vi "SendDrivingCAN.vi"(8 "error in (no error)":errorcluster, 11 "interface object in":refnum<k20>) -> (0 "error out":errorcluster, 3 "interface object out":refnum<k20>)   [LabVIEW 2014]
uses:
  <vilib>/RioEmbeddedCAN/RioEmbeddedCAN.llb/CANFrameControl.ctl
  <vilib>/RioEmbeddedCAN/RioEmbeddedCAN.llb/CANWaitTransmitComplete.vi
  Global Data.vi
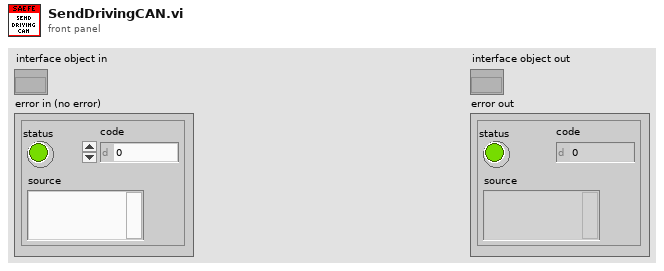
[diagram p1: front panel]
types:
  T1 = typedef "CANFrameControl.ctl" = cluster{"identifier":u32, "extended?":bool, "type":u8, "payload":u8[]}
  T2 = typedef "Lap Statistics.ctl" = cluster{"rBrakeBalLast":dbl}
  T3 = typedef "MC Temp 2.ctl" = cluster{"TMCControlBoard":dbl, "TMCRTD1":dbl, "TMCRTD2":dbl, "TMCRTD3":dbl}
  T4 = typedef "BMS Telemetry.ctl" = cluster{"bBMSIgnition":bool, "bBMSChargerMains":bool, "bBMSFastCharge":bool, "bBMSChargerEnabled":bool, "eBMSCarState":enum16{"Off", "On, Not Charging", "Charging", "Charging Finished", "Charging Error"}, "eBMSChargingState":enum16{"Disconnected", "Pre-charging", "Main Charging", "Balancing", "Charging Finished OK", "Charging Error"}, "tBMSChargeStage":u16, "eBMSLastChargeError":enum16{"No Error", "No Cell Communication", "No Cell Communication - Non CAN Charger", "Maximum charging stage duration expired", "Cell Communication Lost during Charge", "Cannot set balancing voltage", "Cell temps too high", "No Comms so can't determine temp", "# of Cells Mismatch", "Cells Overvoltage", "Cell Protection Event occured."}, "NBMSNumCells":u8, "bBMSUnderVProtection":bool, "bBMSOverVProtection":bool, "bBMSOverTProtection":bool, "bBMSLeakageProtection":bool, "bBMSNoCellCommsError":bool, "bBMSLowVReduction":bool, "bBMSHighTReduction":bool, "VCellMin":dbl, "VCellMax":dbl, "VCellMean":dbl, "VTotal":dbl, "TCellMin":dbl, "TCellMax":dbl, "TCellMean":dbl, "VCells":cluster{"[51]":dbl, "[52]":dbl, "[53]":dbl, "[54]":dbl, "[55]":dbl, "[56]":dbl, "[57]":dbl, "[58]":dbl, "[59]":dbl, "[60]":dbl, "[61]":dbl, "[62]":dbl, "[63]":dbl, "[64]":dbl, "[65]":dbl, "[66]":dbl, "[67]":dbl, "[34]":dbl, "[35]":dbl, "[36]":dbl, "[37]":dbl, "[38]":dbl, "[39]":dbl, "[40]":dbl, "[41]":dbl, "[42]":dbl, "[43]":dbl, "[44]":dbl, "[45]":dbl, "[46]":dbl, "[47]":dbl, "[48]":dbl, "[49]":dbl, "[50]":dbl, "[17]":dbl, "[18]":dbl, "[19]":dbl, "[20]":dbl, "[21]":dbl, "[22]":dbl, "[23]":dbl, "[24]":dbl, "[25]":dbl, "[26]":dbl, "[27]":dbl, "[28]":dbl, "[29]":dbl, "[30]":dbl, "[31]":dbl, "[32]":dbl, "[33]":dbl, "[0]":dbl, "[1]":dbl, "[2]":dbl, "[3]":dbl, "[4]":dbl, "[5]":dbl, "[6]":dbl, "[7]":dbl, "[8]":dbl, "[9]":dbl, "[10]":dbl, "[11]":dbl, "[12]":dbl, "[13]":dbl, "[14]":dbl, "[15]":dbl, "[16]":dbl}, "TCells":cluster{"[55]":dbl, "[56]":dbl, "[57]":dbl, "[58]":dbl, "[59]":dbl, "[60]":dbl, "[61]":dbl, "[62]":dbl, "[63]":dbl, "[64]":dbl, "[65]":dbl, "[66]":dbl, "[67]":dbl, "[68]":dbl, "[69]":dbl, "[70]":dbl, "[17]":dbl, "[38]":dbl, "[39]":dbl, "[40]":dbl, "[41]":dbl, "[42]":dbl, "[43]":dbl, "[44]":dbl, "[45]":dbl, "[46]":dbl, "[47]":dbl, "[48]":dbl, "[49]":dbl, "[50]":dbl, "[51]":dbl, "[52]":dbl, "[53]":dbl, "[54]":dbl, "[21]":dbl, "[22]":dbl, "[23]":dbl, "[24]":dbl, "[25]":dbl, "[26]":dbl, "[27]":dbl, "[28]":dbl, "[29]":dbl, "[30]":dbl, "[31]":dbl, "[32]":dbl, "[33]":dbl, "[34]":dbl, "[35]":dbl, "[36]":dbl, "[37]":dbl, "[0]":dbl, "[1]":dbl, "[2]":dbl, "[3]":dbl, "[4]":dbl, "[5]":dbl, "[6]":dbl, "[7]":dbl, "[8]":dbl, "[9]":dbl, "[10]":dbl, "[11]":dbl, "[12]":dbl, "[13]":dbl, "[14]":dbl, "[15]":dbl, "[16]":dbl}, "bChargerConnected":bool, "VChargerSetpoint":dbl, "IChargerSetpoint":dbl, "VChargerActual":dbl, "IChargerActual":dbl, "BCells":cluster{"[51]":dbl, "[52]":dbl, "[53]":dbl, "[54]":dbl, "[55]":dbl, "[56]":dbl, "[57]":dbl, "[58]":dbl, "[59]":dbl, "[60]":dbl, "[61]":dbl, "[62]":dbl, "[63]":dbl, "[64]":dbl, "[65]":dbl, "[66]":dbl, "[67]":dbl, "[34]":dbl, "[35]":dbl, "[36]":dbl, "[37]":dbl, "[38]":dbl, "[39]":dbl, "[40]":dbl, "[41]":dbl, "[42]":dbl, "[43]":dbl, "[44]":dbl, "[45]":dbl, "[46]":dbl, "[47]":dbl, "[48]":dbl, "[49]":dbl, "[50]":dbl, "[17]":dbl, "[18]":dbl, "[19]":dbl, "[20]":dbl, "[21]":dbl, "[22]":dbl, "[23]":dbl, "[24]":dbl, "[25]":dbl, "[26]":dbl, "[27]":dbl, "[28]":dbl, "[29]":dbl, "[30]":dbl, "[31]":dbl, "[32]":dbl, "[33]":dbl, "[0]":dbl, "[1]":dbl, "[2]":dbl, "[3]":dbl, "[4]":dbl, "[5]":dbl, "[6]":dbl, "[7]":dbl, "[8]":dbl, "[9]":dbl, "[10]":dbl, "[11]":dbl, "[12]":dbl, "[13]":dbl, "[14]":dbl, "[15]":dbl, "[16]":dbl}}
  T5 = typedef "MC Temp 1.ctl" = cluster{"TMCModuleA":dbl, "TMCModuleB":dbl, "TMCModuleC":dbl, "TMCGateDriver":dbl}
  T6 = typedef "MC Temp 3.ctl" = cluster{"TMCRTD4":dbl, "TMCRTD5":dbl, "TMotor":dbl, "MTorqueShudder":dbl}
  T7 = typedef "FPGA Telemetry.ctl" = cluster{"CPU Load":cluster{"Total (%)":dbl, "Time Critical (%)":dbl, "Timed Structures (%)":dbl, "High (%)":dbl, "Above Normal (%)":dbl, "Normal (%)":dbl, "Background (%)":dbl, "Idle (%)":dbl, "ISR (%)":dbl}, "SVehicleStatus":cluster{"BMS Status":T8, "MC Status":T8, "Shutdown Status":T8, "sbRIO Status":T8, "Vehicle Status":T8, "Shutdown State":enum16{"NI.SC.Initial", "NI.SC.History", "NI.SC.ShallowHistory", "NI.SC.Terminal", "Coolant Pump Started/AIR's On", "AIRs On", "Precharge", "TSMS Off"}, "AIR Status":T11, "Remote Return to Pits":bool, "Reason for Shutdown":T12, "MC State Machine Status":enum16{"NI.SC.Initial", "NI.SC.History", "NI.SC.ShallowHistory", "NI.SC.Terminal", "Broadcast Diag", "Let Current Drop then Disable AIR's", "Enabled", "Disabled"}}, "iPhone HF Data":cluster{"gXiPhone":dbl, "gYiPhone":dbl, "gZiPhone":dbl, "nYawXiPhone":dbl, "nYawYiPhone":dbl, "nYawZiPhone":dbl}, "iPhone LF Data":cluster{"nLatiPhone":dbl, "nLongiPhone":dbl, "nGPSiPhone":dbl}, "stop":bool, "VSupplyOffset":fxp<+,12,4>, "VsbRIOSupply":fxp<+/-,25,6>, "bFPGALED":bool, "TSBRIO":fxp<+/-,33,17>, "rTPS2Unscaled":fxp<+/-,16,1>, "rTPS1Unscaled":fxp<+/-,16,1>, "bTPSConsistent":bool, "bTPSInRange":bool, "rThrottle":fxp<+/-,33,22>, "VTPS2":fxp<+/-,24,5>, "rTPS2":fxp<+/-,31,22>, "VTPS1":fxp<+/-,24,5>, "rTPS1":fxp<+/-,31,22>, "rTPS2Max":fxp<+,16,4>, "rTPS2Min":fxp<+,16,4>, "rTPS1Max":fxp<+,16,4>, "rTPS1Min":fxp<+,16,4>, "bCoolantPumpEnable":bool, "bRTDSEnable":bool, "bTSMSInStatus":bool, "bPosAIREnable":bool, "bBMSOK":bool, "bIMDOK":bool, "bBSPDOK":bool, "bSBRIOOK2":bool, "bSBRIOOK1":bool, "bTSMSOutStatus":bool, "eGreenDash":T13, "eYellowDash":T13, "eRedDash":T13, "bMotorControllerEnable":bool, "tCurrentLap":u32, "bNewLap":bool, "tLastLap":u32, "tLapMin":u32, "V5VSupply":fxp<+/-,24,5>, "bWheelRL":bool, "bWheelRR":bool, "bWheelFR":bool, "bWheelFL":bool, "VBrakePressureR":fxp<+/-,24,5>, "VBrakePressureF":fxp<+/-,24,5>, "bWheelRRStopped":bool, "bWheelRLStopped":bool, "bWheelFRStopped":bool, "bWheelFLStopped":bool, "tWheelRLPeriod":u32, "tWheelRRPeriod":u32, "tWheelFRPeriod":u32, "tWheelFLPeriod":u32, "bBrakeLight":bool, "VShockRR":fxp<+/-,24,5>, "VShockRL":fxp<+/-,24,5>, "VShockFR":fxp<+/-,24,5>, "VShockFL":fxp<+/-,24,5>, "IHighCurrent":fxp<+/-,24,15>, "ILowCurrent":fxp<+/-,24,15>, "pBrakeR":fxp<+,26,13>, "pBrakeF":fxp<+,26,13>, "bHighCurrentOK":bool, "bLowCurrentOK":bool, "bBrakeROK":bool, "bBrakeFOK":bool, "VSteerWheelMiddle":fxp<+/-,26,5>, "aSteerWheel":fxp<+/-,31,13>, "nWheelFL":fxp<+/-,32,16>, "nWheelFR":fxp<+/-,32,16>, "nWheelRL":fxp<+/-,32,16>, "nWheelRR":fxp<+/-,32,16>, "ADXL345 Output":T14, "Tire Diameter(m)":fxp<+,16,1>, "vWheelRR":fxp<+/-,32,18>, "vWheelRL":fxp<+/-,32,18>, "vWheelFR":fxp<+/-,32,18>, "vWheelFL":fxp<+/-,32,18>, "vWheelLowest":fxp<+/-,32,18>, "vWheelHighest":fxp<+/-,32,18>, "bAccel":bool, "vAxleF":fxp<+/-,33,19>, "vCar":fxp<+/-,33,19>, "sLap":fxp<+,32,12>, "rSlipRL":fxp<+/-,12,1>, "rSlipRR":fxp<+/-,12,1>, "rSlipFL":fxp<+/-,12,1>, "rSlipFR":fxp<+/-,12,1>, "NLap":u8, "tLapReference":u32, "tFastestLap":u32, "MTorqueRequest":dbl, "RS232 Error Out":cluster{"status":bool, "code":i32}}
  T8 = typedef "Subsystem Status.ctl" = cluster{"eStatusSeverity":T9, "NValue":sgl, "CMessage":T10, "bNotOK":bool}
  T9 = typedef "Subsystem Status Severity.ctl" = enum16{"Okay", "Short Warning", "Long Warning", "Return to Pits", "Error", "Danger"}
  T10 = typedef "Subsystem Status Message.ctl" = enum16{"ControllerTemperature", "MotorTemperature", "BatteryTemperature", "BatteryLowVoltage", "LVBattery", "sbRIOTemperature", "Precharge", "BSPD", "IMD", "RemoteReturnToPits", "EStopInterrupted", "NoCellComms", "MCOverSpeed", "MCOverCurrent", "MCOverVoltage", "MCInverterOverTemp", "MCDirectionCommand", "MCInverterTimeout", "MCDesatFault", "MCHWOverCurrent", "MCUnderVoltage", "MCCommandMessageLost", "MotorOverTemp", "MCModAOverTemp", "MCModBOverTemp", "MCModCOverTemp", "MCPCBOverTemp", "MCGateDrv1OverTemp", "MCDateDrv2OverTemp", "MCCurrentSensorFault", "MCResolverNotConnected", "ShutdownLatchTripped", "UnknownBMS", "RemoteEmergency"}
  T11 = typedef "AIR Status.ctl" = enum16{"Off", "Precharge", "On"}
  T12 = typedef "Reason for Shutdown.ctl" = enum16{"None", "BMS", "Shutdown", "sbRIO", "MC", "Remote"}
  T13 = typedef "Dash LED Status.ctl" = enum16{"Off", "Flashing", "On"}
  T14 = typedef "ADXL345 Output.ctl" = cluster{"X":fxp<+/-,14,4>, "Y":fxp<+/-,14,4>, "Z":fxp<+/-,14,4>}
  T15 = typedef "Shutdown State Machine.lvsc/State.ctl" = enum16{"NI.SC.Initial", "NI.SC.History", "NI.SC.ShallowHistory", "NI.SC.Terminal", "Coolant Pump Started/AIR's On", "AIRs On", "Precharge", "TSMS Off"}
  T16 = typedef "MC State Machine.lvsc/State.ctl" = enum16{"NI.SC.Initial", "NI.SC.History", "NI.SC.ShallowHistory", "NI.SC.Terminal", "Broadcast Diag", "Let Current Drop then Disable AIR's", "Enabled", "Disabled"}
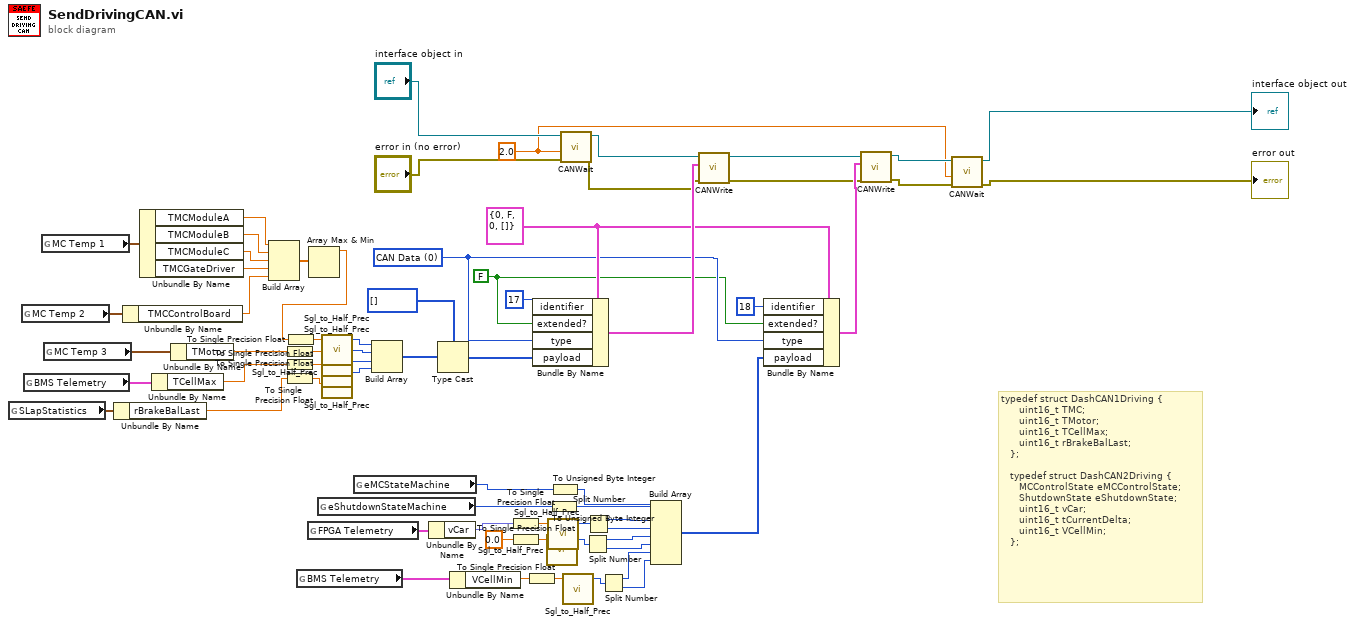
[diagram p0: block diagram]
diagram:
  w6 = 2.0 ("timeout (0 s)")
  w61 = u8 0 items=["CAN Data", "CAN Remote"] ("type")
  w63 = T1 {"identifier"=0, "extended?"=FALSE, "type"=0, "payload"=[]} ("CAN frame")
  w60 = FALSE ("extended?")
  # "typedef struct DashCAN1Driving {\n      uint16_t TMC;\n      uint16_t TMotor;\n      uint16_t TCellMax;\n      uint16_t rBrakeBalLast;\n   };\n\n   typedef struct DashCAN2Driving {\n      MCControlState eMCControlState;\n      ShutdownState eShutdownState;\n      uint16_t vCar;\n      uint16_t tCurrentDelta;\n      uint16_t VCellMin;\n   };"
  n1 = global read "Global Data.vi" "SLapStatistics"() -> (w21:T2)
  n2 = global read "Global Data.vi" "MC Temp 2"() -> (w48:T3)
  n3 = global read "Global Data.vi" "BMS Telemetry"() -> (w39:T4)
  n4 = global read "Global Data.vi" "MC Temp 1"() -> (w49:T5)
  n5 = global read "Global Data.vi" "MC Temp 3"() -> (w52:T6)
  n6 = Unbundle By Name(w21) -> ("rBrakeBalLast"=w19:dbl)
  n7 = Unbundle By Name(w48) -> ("TMCControlBoard"=w43:dbl)
  n8 = Unbundle By Name(w49) -> ("TMCModuleA"=w47:dbl, "TMCModuleB"=w46:dbl, "TMCModuleC"=w45:dbl, "TMCGateDriver"=w44:dbl)
  n9 = Unbundle By Name(w39) -> ("TCellMax"=w37:dbl)
  n10 = Unbundle By Name(w52) -> ("TMotor"=w51:dbl)
  n11 = Build Array(w47, w46, w45, w44, w43) -> (w42:dbl[])
  n12 = To Single Precision Float(number=w51) -> (single precision float=w50:sgl)
  n13 = To Single Precision Float(number=w37) -> (single precision float=w38:sgl)
  n14 = To Single Precision Float(number=w19) -> (single precision float=w20:sgl)
  n15 = global read "Global Data.vi" "BMS Telemetry"() -> (w17:T4)
  n16 = global read "Global Data.vi" "FPGA Telemetry"() -> (w23:T7)
  n17 = Array Max & Min(array=w42) -> (max value=w40:dbl)  [unwired: 3 out]
  n18 = To Single Precision Float(number=w40) -> (single precision float=w41:sgl)
  n19 = global read "Global Data.vi" "eShutdownStateMachine"() -> (w24:T15)
  n20 = call "Sgl_to_Half_Prec.vi"("SGL"=w41) -> ("Half Precision Floating Point"=w56:u16)  [unwired: 4 in]
  n21 = call "Sgl_to_Half_Prec.vi"("SGL"=w50) -> ("Half Precision Floating Point"=w55:u16)  [unwired: 4 in]
  n22 = call "Sgl_to_Half_Prec.vi"("SGL"=w38) -> ("Half Precision Floating Point"=w54:u16)  [unwired: 4 in]
  n23 = call "Sgl_to_Half_Prec.vi"("SGL"=w20) -> ("Half Precision Floating Point"=w53:u16)  [unwired: 4 in]
  n24 = global read "Global Data.vi" "eMCStateMachine"() -> (w25:T16)
  n25 = Build Array(w56, w55, w54, w53) -> (w57:u16[])
  n26 = Unbundle By Name(w23) -> ("vCar"=w22:fxp<+/-,33,19>)
  n27 = Type Cast(type=u8[] [], x=w57) -> (*(type *) &x=w59:u8[])
  n28 = Unbundle By Name(w17) -> ("VCellMin"=w14:dbl)
  n29 = To Single Precision Float(number=w22) -> (single precision float=w36:sgl)
  n30 = To Single Precision Float(number=sgl 0.0) -> (single precision float=w35:sgl)
  n31 = To Single Precision Float(number=w14) -> (single precision float=w16:sgl)
  n32 = Bundle By Name(cluster=w63, "identifier"=u32 17, "extended?"=w60, "type"=w61, "payload"=w59) -> (w65:T1)
  n33 = call "Sgl_to_Half_Prec.vi"("SGL"=w35) -> ("Half Precision Floating Point"=w34:u16)  [unwired: 4 in]
  n34 = call "Sgl_to_Half_Prec.vi"("SGL"=w36) -> ("Half Precision Floating Point"=w33:u16)  [unwired: 4 in]
  n35 = To Unsigned Byte Integer(number=w24) -> (unsigned 8bit integer=w31:u8)
  n36 = To Unsigned Byte Integer(number=w25) -> (unsigned 8bit integer=w32:u8)
  n37 = call-poly <vilib>:"CANWait.vi"("error in (no error)"="error in (no error)", "timeout (0 s)"=w6, "interface object in"="interface object in") -> ("error out"=w8:errorcluster, "interface object out"=w9:refnum<k20>)  [unwired: 7 in]
  n38 = call "Sgl_to_Half_Prec.vi"("SGL"=w16) -> ("Half Precision Floating Point"=w15:u16)  [unwired: 4 in]
  n39 = Split Number(x=w34) -> (hi(x)=w28:u8, lo(x)=w27:u8)
  n40 = Split Number(x=w33) -> (hi(x)=w30:u8, lo(x)=w29:u8)
  n41 = Split Number(x=w15) -> (hi(x)=w13:u8, lo(x)=w12:u8)
  n42 = Build Array(w32, w31, w30, w29, w28, w27, w13, w12) -> (w26:u8[])
  n43 = call <vilib>:"CANWrite.vi"("error in (no error)"=w8, "CAN frame"=w65, "interface object in"=w9) -> ("error out"=w3:errorcluster, "interface object out"=w4:refnum<k20>)  [unwired: 7 in]
  n44 = Bundle By Name(cluster=w63, "identifier"=u32 18, "extended?"=w60, "type"=w61, "payload"=w26) -> (w64:T1)
  n45 = call <vilib>:"CANWrite.vi"("error in (no error)"=w3, "CAN frame"=w64, "interface object in"=w4) -> ("error out"=w5:errorcluster, "interface object out"=w7:refnum<k20>)  [unwired: 7 in]
  n46 = call-poly <vilib>:"CANWait.vi"("error in (no error)"=w5, "timeout (0 s)"=w6, "interface object in"=w7) -> ("error out"=→"error out":errorcluster, "interface object out"=→"interface object out":refnum<k20>)  [unwired: 7 in]
